vi "ex_GetAllExpressAttribs.vi"(8 "error in":errorcluster, 11 "Signals":waveform(dbl)[](array[waveform])) -> (0 "error out":errorcluster, 1 "All Express Wave Attributes":T1(array[cluster]) {"Timestamp" format="%<%X\n%x>T"; "Start Timestamp" format="%<%X\n%x>T"})   [LabVIEW 2017]
uses:
  <vilib>/express/express shared/transition.llb/ex_WaveformAttribs.ctl
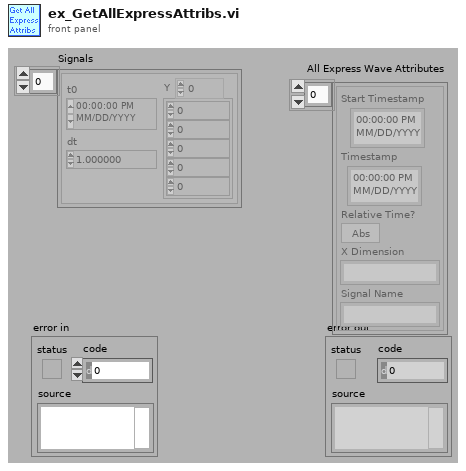
[diagram p1: front panel]
types:
  T1 = cluster{"Start Timestamp":timestamp, "Timestamp":timestamp, "Relative Time?":bool, "X Dimension":string, "Signal Name":string}[]
  T2 = typedef "ex_WaveformAttribs.ctl" = cluster{"Start Timestamp":timestamp, "Timestamp":timestamp, "Relative Time?":bool, "X Dimension":string, "Signal Name":string}
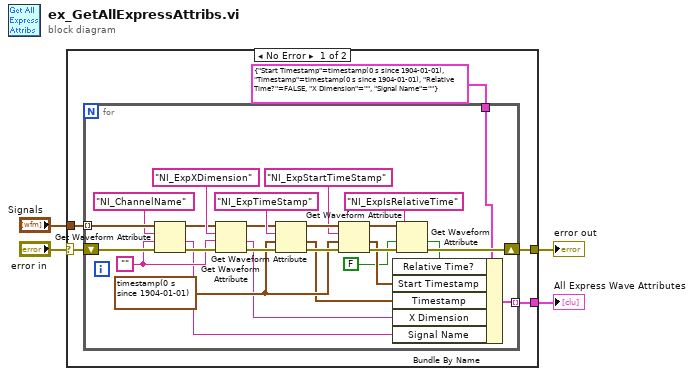
[diagram p0: block diagram]
diagram:
  n1 = case shown="No Error" "error in" {
    selector: "error in" -> [w8 w36]
    tunnel: [w9 w36] -> w4
    tunnel: "Signals" -> [w7 _]
    tunnel: [w6 _] -> w2
    frame No Error {
      n2 = for {
        tunnel: w7 -> [w26] mode=indexing
        shift-right: [w27] -> w9
        shift-left: w8 -> [w25]
        tunnel: [w10] -> w6 mode=indexing
        tunnel: T2 {"Start Timestamp"=timestamp(0 s since 1904-01-01), "Timestamp"=timestamp(0 s since 1904-01-01), "Relative Time?"=FALSE, "X Dimension"="", "Signal Name"=""} ("All Express Wave Attributes 2") -> [w19]
        w16 = ""
        w17 = timestamp(0 s since 1904-01-01)
        n3 = Get Waveform Attribute(4:w25, 5:w16, 6:"NI_ChannelName" ("name"), 7:w26) -> (0:w22:errorcluster, 1:w13:string, 3:w23:waveform(dbl))  [unwired: 1 out]
        n4 = Get Waveform Attribute(4:w22, 5:w16, 6:"NI_ExpXDimension" ("name"), 7:w23) -> (0:w20:errorcluster, 1:w12:string, 3:w21:waveform(dbl))  [unwired: 1 out]
        n5 = Get Waveform Attribute(4:w20, 5:w17, 6:"NI_ExpTimeStamp" ("name"), 7:w21) -> (0:w31:errorcluster, 1:w14:timestamp, 3:w32:waveform(dbl))  [unwired: 1 out]
        n6 = Get Waveform Attribute(4:w31, 5:w17, 6:"NI_ExpStartTimeStamp" ("name"), 7:w32) -> (0:w34:errorcluster, 1:w18:timestamp, 3:w35:waveform(dbl))  [unwired: 1 out]
        n7 = Get Waveform Attribute(4:w34, 5:FALSE, 6:"NI_ExpIsRelativeTime" ("name"), 7:w35) -> (0:w27:errorcluster, 1:w11:bool)  [unwired: 2 out]
        n8 = Bundle By Name(cluster=w19, "Relative Time?"=w11, "Start Timestamp"=w18, "Timestamp"=w14, "X Dimension"=w12, "Signal Name"=w13) -> (w10:T2)
      }
    }
    frame Error {
    }
  }
  "error out" <- w4
  "All Express Wave Attributes" <- w2
